vi "Save Yaml.vi"(8 "error in (no error)":errorcluster, 11 "Yaml Model in":refnum<class "Yaml Model.lvclass">) -> (0 "error out":errorcluster, 3 "Yaml Model out":refnum<class "Yaml Model.lvclass">)   [LabVIEW 2020, in "Yaml Model.lvlib" / "Yaml Model.lvclass"]
uses:
  Yaml Model.lvclass
  Yaml Model.lvclass/Yaml Model.ctl
panel:
  # "NOTICE -- YOU MUST LEAVE THIS NOTICE IN PLACE.\n\nCopyright (c) 2017, LIANG LIU Shawn.Liu.cn@gmail.com\nAll rights reserved.\n\nRedistribution and use in source and binary forms, with or without modification, are permitted provided that the following conditions are met:\n-Redistributions of source code must retain the above copyright notice, this list of conditions and the following disclaimer.\n-Redistributions in binary form must reproduce the above copyright notice, this list of conditions and the following disclaimer in the documentation and/or other materials provided with the distribution.\n-Neither the name of the eLp nor the names of its contributors may be used to endorse or promote products derived from this software without specific prior written permission.\n\nTHIS SOFTWARE IS PROVIDED BY THE COPYRIGHT HOLDERS AND CONTRIBUTORS \"AS IS\" AND ANY EXPRESS OR IMPLIED WARRANTIES, INCLUDING, BUT NOT LIMITED TO, THE IMPLIED WARRANTIES OF MERCHANTABILITY AND FITNESS FOR A PARTICULAR PURPOSE ARE DISCLAIMED. IN NO EVENT SHALL THE COPYRIGHT HOLDER OR CONTRIBUTORS BE LIABLE FOR ANY DIRECT, INDIRECT, INCIDENTAL, SPECIAL, EXEMPLARY, OR CONSEQUENTIAL DAMAGES (INCLUDING, BUT NOT LIMITED TO, PROCUREMENT OF SUBSTITUTE GOODS OR SERVICES; LOSS OF USE, DATA, OR PROFITS; OR BUSINESS INTERRUPTION) HOWEVER CAUSED AND ON ANY THEORY OF LIABILITY, WHETHER IN CONTRACT, STRICT LIABILITY, OR TORT (INCLUDING NEGLIGENCE OR OTHERWISE) ARISING IN ANY WAY OUT OF THE USE OF THIS SOFTWARE, EVEN IF ADVISED OF THE POSSIBILITY OF SUCH DAMAGE."
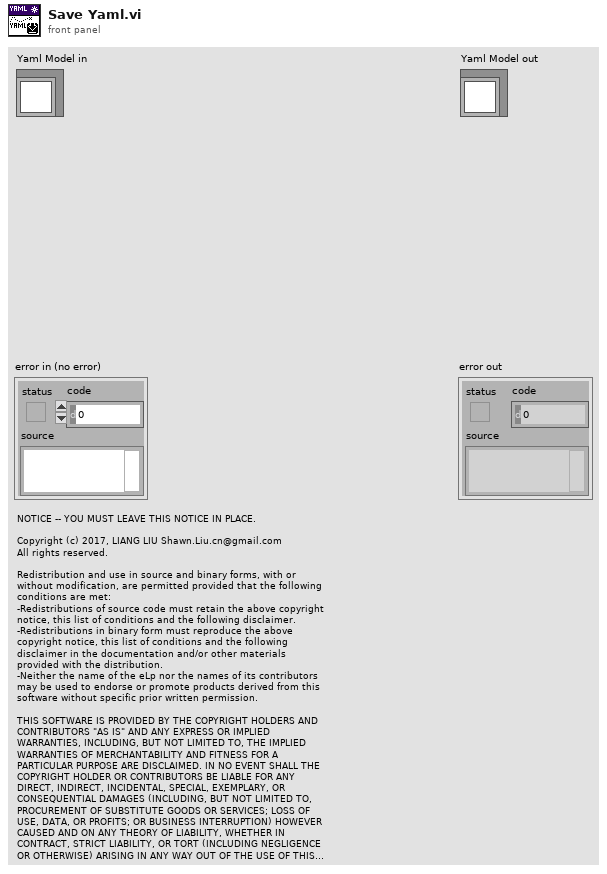
[diagram p1: front panel]
types:
  T1 = enum8{"Enabled", "Disabled", "Disabled and Grayed Out"}
  T2 = enum16{"open", "replace", "create", "open or create", "replace or create", "replace or create with confirmation"}
  T3 = cluster{"Image":string, "Resolution":dbl, "Origin":cluster{"X":dbl, "Y":dbl, "R":dbl}, "Occupied Thresh":dbl, "Free Thresh":dbl, "Negate":bool}
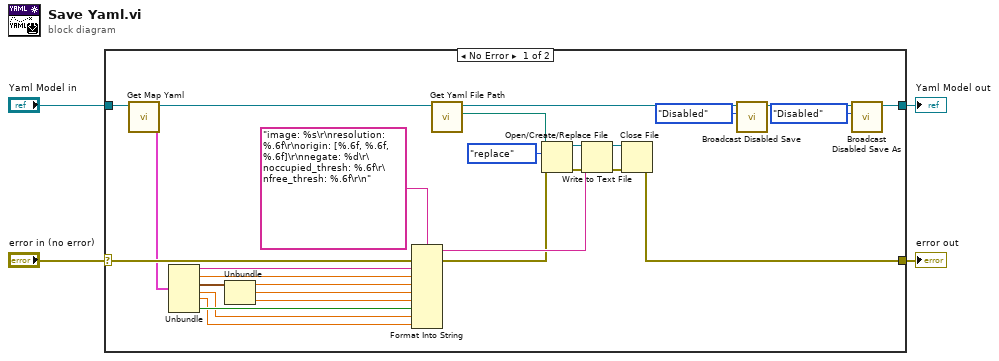
[diagram p0: block diagram]
diagram:
  n1 = case shown="No Error" "error in (no error)" {
    selector: "error in (no error)" -> [w29 w34]
    tunnel: "Yaml Model in" -> [w32 w33]
    tunnel: [w30 w34] -> w3
    tunnel: [w7 w33] -> w1
    frame No Error {
      n2 = call "Get Map Yaml.vi"("Yaml Model in"=w32) -> ("Map Yaml"=w26:T3, "Yaml Model out"=w28:refnum<class "Yaml Model.lvclass">)  [unwired: 9 in]
      n3 = Unbundle(w26) -> ("Image"=w25:string, "Resolution"=w24:dbl, "Origin"=w20:cluster{"X":dbl, "Y":dbl, "R":dbl}, "Occupied Thresh"=w18:dbl, "Free Thresh"=w17:dbl, "Negate"=w19:bool)
      n4 = Unbundle(w20) -> ("X"=w23:dbl, "Y"=w22:dbl, "R"=w21:dbl)
      n5 = Format Into String(format string="image: %s\r\nresolution: %.6f\r\norigin: [%.6f, %.6f, %.6f]\r\nnegate: %d\r\noccupied_thresh: %.6f\r\nfree_thresh: %.6f\r\n", error in=w29, w25, w24, w23, w22, w21, w19, w18, w17) -> (resulting string=w12:string, error out=w10:errorcluster)  [unwired: 1 in]
      n6 = call "Get Yaml File Path.vi"("Yaml Model in"=w28) -> ("Yaml File Path"=w9:path, "Yaml Model out"=w31:refnum<class "Yaml Model.lvclass">)  [unwired: 9 in]
      n7 = Open/Create/Replace File(file path (use dialog)=w9, error in=w10, operation (0:open)=T2."replace") -> (refnum out=w16:refnum<file>, error out=w15:errorcluster)  [unwired: 3 in, 1 out]
      n8 = Write to Text File(file (use dialog)=w16, text=w12, error in=w15) -> (refnum out=w14:refnum<file>, error out=w13:errorcluster)  [unwired: 1 in, 1 out]
      n9 = Close File(refnum=w14, error in=w13) -> (error out=w30:errorcluster)  [unwired: 1 out]
      n10 = call "Broadcast Disabled Save.vi"("Disabled Save"=T1."Disabled", "Yaml Model in"=w31) -> ("Yaml Model out"=w8:refnum<class "Yaml Model.lvclass">)  [unwired: 8 in, 1 out]
      n11 = call "Broadcast Disabled Save As.vi"("Disabled Save As"=T1."Disabled", "Yaml Model in"=w8) -> ("Yaml Model out"=w7:refnum<class "Yaml Model.lvclass">)  [unwired: 8 in, 1 out]
    }
    frame Error {
    }
  }
  "error out" <- w3
  "Yaml Model out" <- w1
